vi "Channel Probe.vi"(2 "channelOp":T1, 3 "data in":refnum<class "EventMessengerData.lvclass">) -> (1 "data out":refnum<class "EventMessengerData.lvclass">)   [LabVIEW 2019, in "Cmd-Data Event Messenger.lvlib"]
doc: "Displays the status of the channel as the channel is modified by the various endpoints and gives the user ways to pause the application using the channel."
uses:
  Cmd-Data Event Messenger.lvlib
  EventMessengerData.lvclass
  ChannelOp.ctl
panel:
  out "High Priority?":bool
  in  "Details":string="Details"
  in  "Write Count":string="Write Count"
  out "Details":string
  in  "Pause when aborted":bool
  in  "Pause when last element written":bool
  out "Details":string
  in  "Play":bool
  out "Aborted?":bool
  out "Last element written?":bool
  in  "Pause":bool
  # "Details"
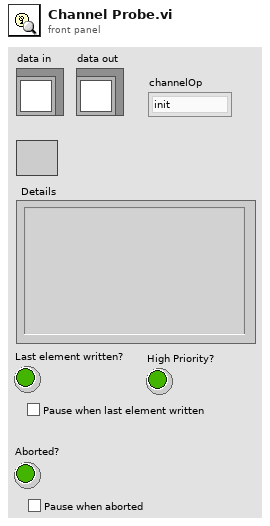
[diagram p1: front panel]
types:
  T1 = typedef "Cmd-Data Event Messenger.lvlib/ChannelOp.ctl" = enum16{"init", "write", "register", "replicate", "probe"}
  T2 = enum32{"Invalid", "Standard", "Closed", "Hidden", "Minimized", "Maximized"}
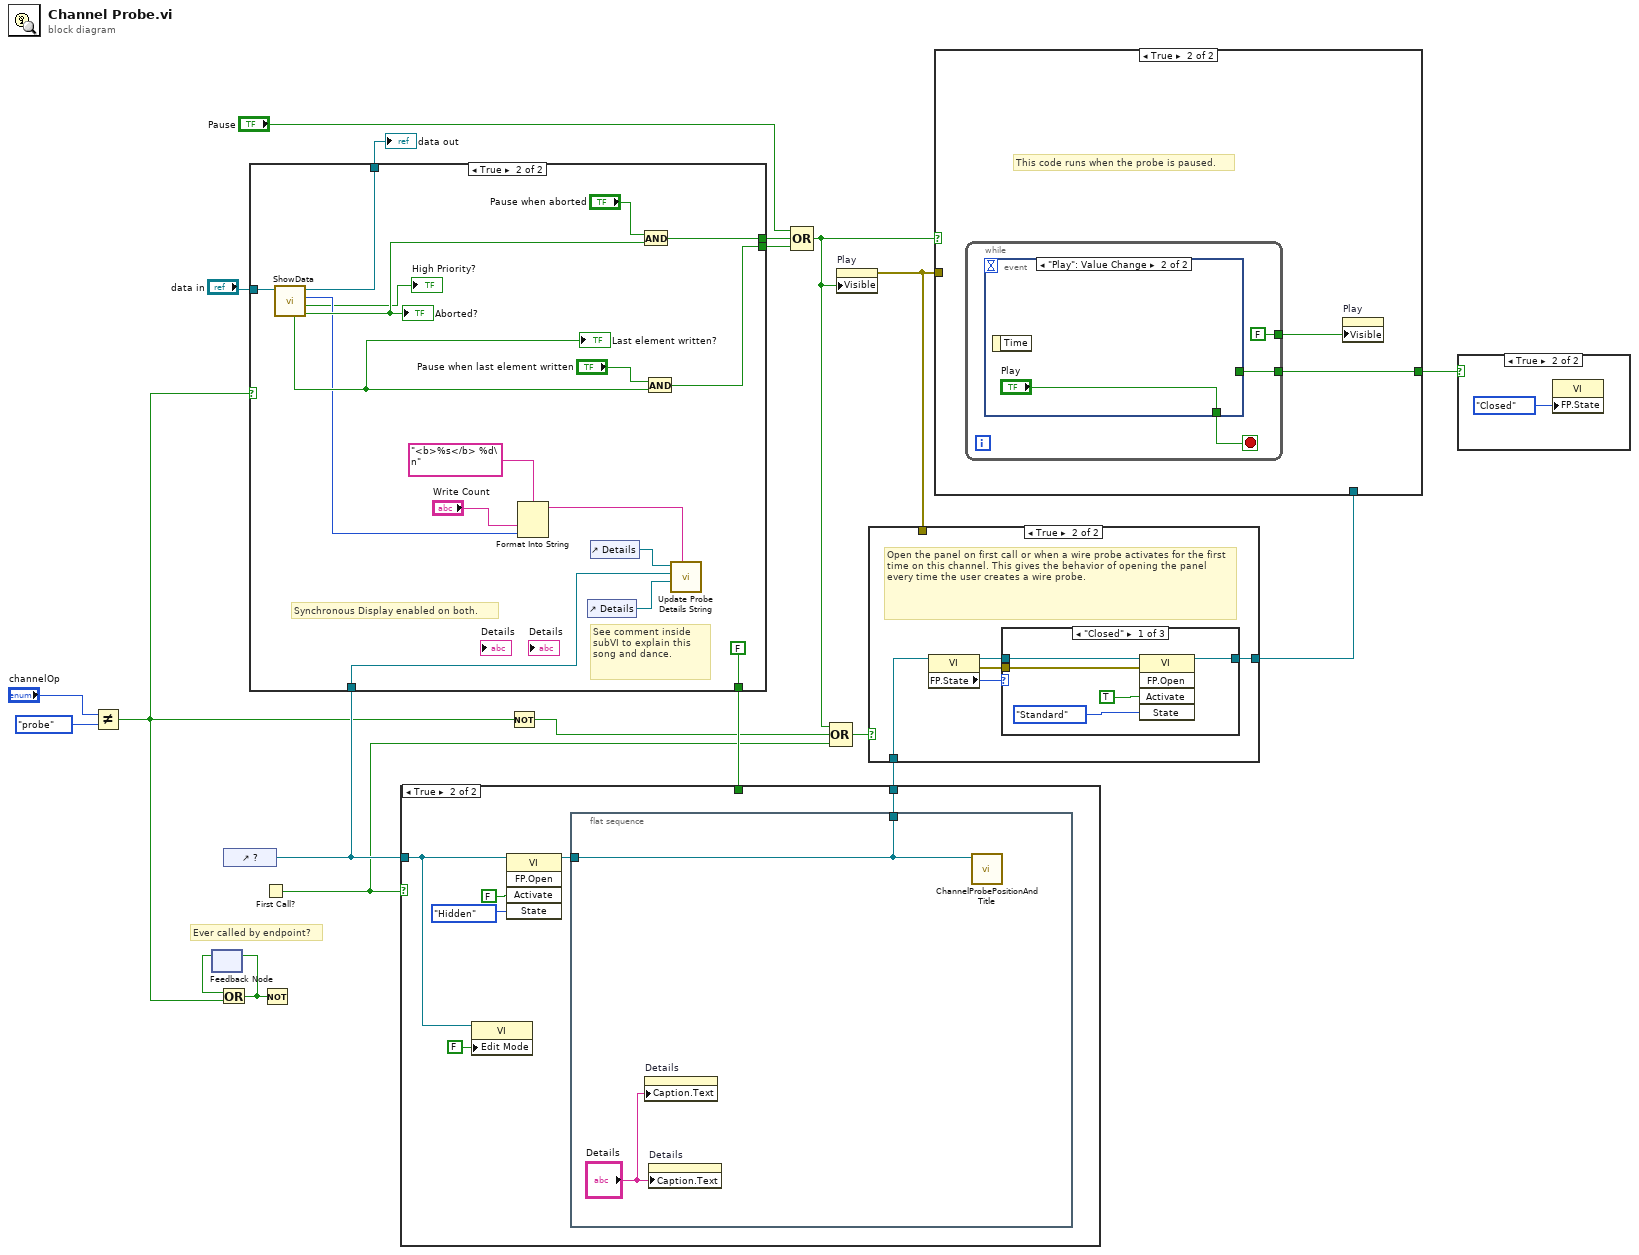
[diagram p0: block diagram]
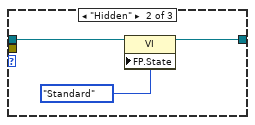
[diagram p3: hidden frame]
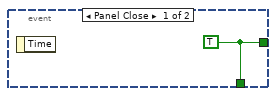
[diagram p8: hidden frame]
diagram:
  # "Ever called by endpoint?"
  n1 = Not Equal?(x="channelOp", y=ChannelOp."probe" ("channelOp")) -> (x != y?=w1:bool)
  n2 = feedback #1() -> (w13:bool)  [unwired: 1 in]
  n3 = Or(x=w13, y=w1) -> (x .or. y?=w12:bool)
  n4 = feedback-in #1(w12) -> ()
  n5 = control-ref of="?"() -> (w14:refnum<vi>)
  n6 = case shown="True" w1 {
    tunnel: "data in" -> [w21 w38]
    tunnel: [_ w35] -> w18
    tunnel: [_ w34] -> w16
    tunnel: [_ FALSE ("always false")] -> w15
    tunnel: w14 -> [_ w32]
    tunnel: [w21 w27] -> w3
    frame False {
    }
    frame True {
      # "See comment inside subVI to explain this song and dance."
      # "Synchronous Display enabled on both."
      n7 = call "ShowData.vi"("data in"=w38) -> ("aborted?"=w25:bool, "high priority?"=→"High Priority?":bool, "write count"=w24:u32, "data out"=w27:refnum<class "EventMessengerData.lvclass">, "last element?"=w26:bool)  [unwired: 6 in]
      "Last element written?" <- w26
      "Aborted?" <- w25
      n8 = Format Into String(format string="<b>%s</b> %d\n", "Write Count", w24) -> (resulting string=w23:string)  [unwired: 2 in, 1 out]
      n9 = control-ref of="Details"() -> (w33:refnum<vi>)
      n10 = control-ref of="Details"() -> (w31:refnum<vi>)
      n11 = And(x="Pause when aborted", y=w25) -> (x .and. y?=w35:bool)
      n12 = And(x="Pause when last element written", y=w26) -> (x .and. y?=w34:bool)
      n13 = call <resource>:"Update Probe Details String.vi"("String"=w23, "Details 1"=w33, "VI Reference"=w32, "Details 2"=w31) -> ()  [unwired: 8 in]
    }
  }
  "data out" <- w3
  n14 = First Call?() -> (First Call?: T/F=w5:bool)
  n15 = Not(x=w12) -> ()  [unwired: 1 out]
  n16 = case shown="True" w5 {
    tunnel: [w39 w45] -> w10
    tunnel: w14 -> [w39 w41]
    tunnel: w15 -> [_ _]
    frame False {
    }
    frame True {
      n17 = property class="VI"(reference=w41, "Edit Mode"=FALSE ("Edit Mode On Open")) -> ()  [unwired: 1 in, 2 out]
      n18 = invoke class="VI" method="FP.Open"(reference=w41, "Activate"=FALSE ("Activate?"), "State"=T2."Hidden") -> (reference out=w42:refnum<vi>)  [unwired: 2 in, 4 out]
      n19 = flat-sequence {
        tunnel: [w46] -> w45
        tunnel: w42 -> [w46]
        frame #0 {
          n20 = property on="Details" class="Str"("Caption.Text"="Details") -> ()  [unwired: 2 in, 2 out]
          n21 = property on="Details" class="Str"("Caption.Text"="Details") -> ()  [unwired: 2 in, 2 out]
          n22 = call <resource>:"ChannelProbePositionAndTitle.vi"("VI in"=w46) -> ()  [unwired: 9 in, 2 out]
        }
      }
    }
  }
  n23 = Not(x=w1) -> (.not. x?=w6:bool)
  n24 = Compound Arithmetic op=OR("Pause", w18, w16) -> (w2:bool)
  n25 = Compound Arithmetic op=OR(w2, w6, w5) -> (w4:bool)
  n26 = property on="Play" class="Bool"("Visible"=w2) -> (error out=w9:errorcluster)  [unwired: 2 in, 1 out]
  n27 = case shown="True" w4 {
    tunnel: [w48 w50] -> w11
    tunnel: w10 -> [w48 w49]
    tunnel: w9 -> [_ _]
    frame False {
    }
    frame True {
      # "Open the panel on first call or when a wire probe activates for the first time on this channel. This gives the behavior of opening the panel every time the user creates a wire probe."
      n28 = property class="VI"(reference=w49) -> (reference out=w51:refnum<vi>, error out=w52:errorcluster, "FP.State"=w53:T2)  [unwired: 1 in]
      n29 = case shown="\"Closed\"" w53 {
        tunnel: w52 -> [w57 _ _]
        tunnel: w51 -> [w58 w61 w62]
        tunnel: [w54 w60 w62] -> w50
        frame "Closed" {
          n30 = invoke class="VI" method="FP.Open"(reference=w58, error in=w57, "Activate"=TRUE ("Activate?"), "State"=T2."Standard") -> (reference out=w54:refnum<vi>)  [unwired: 1 in, 4 out]
        }
        frame "Hidden" {
          n31 = property class="VI"(reference=w61, "FP.State"=T2."Standard" ("Front Panel Window:State")) -> (reference out=w60:refnum<vi>)  [unwired: 1 in, 1 out]
        }
        frame Default {
        }
      }
    }
  }
  n32 = case shown="True" w2 {
    tunnel: w11 -> [_ _]
    tunnel: [_ w64] -> w20
    tunnel: w9 -> [_ _]
    frame False {
    }
    frame True {
      # "This code runs when the probe is paused."
      n33 = while {
        tunnel: [w67] -> w64
        tunnel: [FALSE ("Visible")] -> w63
        stop <- w66 stop-if-true
        n34 = event shown="[1] \"Play\": Value Change" {
          selector: _ -> [_ _]
          dyn-events: _ -> [_ _]
          timeout: _ -> [_ _]
          tunnel: [w68 _] -> w67
          tunnel: [w68 "Play"] -> w66
          event Panel Close {
            w68 = TRUE
            n35 = event-data() -> ()  [unwired: 1 in, 1 out]
          }
          event "Play": Value Change {
            n36 = event-data() -> ()  [unwired: 1 in, 1 out]
          }
        }
      }
      n37 = property on="Play" class="Bool"("Visible"=w63) -> ()  [unwired: 2 in, 2 out]
    }
  }
  n38 = case shown="True" w20 {
    frame False {
    }
    frame True {
      n39 = property class="VI"("FP.State"=T2."Closed" ("Front Panel Window:State")) -> ()  [unwired: 2 in, 2 out]
    }
  }
